vi "2015Swerve.vi"(0 "Axes":dbl[](array[numeric]), 2 "Robot Dimension Calc":dbl, 4 "EncoderTicksPerRev":dbl, 6 "Encoder Offset":dbl) -> (20 "SteeringArray":dbl[](array[numeric]), 22 "PowerArray":dbl[](array[numeric]))   [LabVIEW 2014]
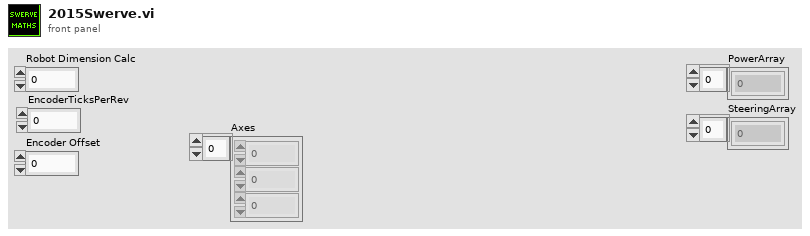
[diagram p1: front panel]
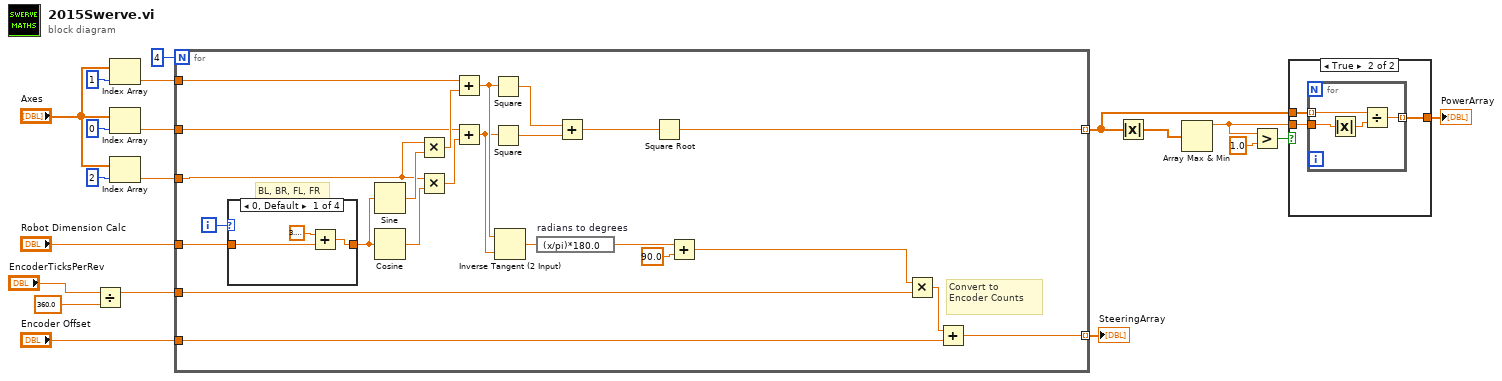
[diagram p0: block diagram]
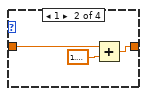
[diagram p3: hidden frame]
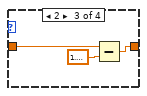
[diagram p4: hidden frame]
diagram:
  n1 = Divide(x="EncoderTicksPerRev", y=360.0) -> (x/y=w5:dbl)
  n2 = Index Array(array="Axes", index=1) -> (element=w9:dbl)
  n3 = Index Array(array="Axes", index=0) -> (element=w10:dbl)
  n4 = Index Array(array="Axes", index=2) -> (element=w11:dbl)
  n5 = for {
    N: 4 -> [_]
    tunnel: "Robot Dimension Calc" -> [w44]
    tunnel: w11 -> [w23]
    tunnel: w10 -> [w22]
    tunnel: w9 -> [w21]
    tunnel: [w27] -> w1 mode=indexing
    tunnel: [w25] -> w15 mode=indexing
    tunnel: w5 -> [w29]
    tunnel: "Encoder Offset" -> [w26]
    i -> [w39]
    # "Convert to\nEncoder Counts"
    # "BL, BR, FL, FR"
    n6 = case shown="0, Default" w39 {
      tunnel: [w46 w50 w53 w54] -> w30
      tunnel: w44 -> [w47 w48 w51 w54]
      frame 0, Default {
        n7 = Add(x=3.141592653589793, y=w47) -> (x+y=w46:dbl)
      }
      frame 1 {
        n8 = Add(x=w48, y=1.5707963267948966) -> (x+y=w50:dbl)
      }
      frame 2 {
        n9 = Subtract(x=w51, y=1.5707963267948966) -> (x-y=w53:dbl)
      }
      frame 3 {
      }
    }
    n10 = Sine(x=w30) -> (sin(x)=w42:dbl)
    n11 = Cosine(x=w30) -> (cos(x)=w43:dbl)
    n12 = Multiply(x=w23, y=w42) -> (x*y=w33:dbl)
    n13 = Multiply(x=w23, y=w43) -> (x*y=w41:dbl)
    n14 = Add(x=w21, y=w33) -> (x+y=w38:dbl)
    n15 = Add(x=w22, y=w41) -> (x+y=w34:dbl)
    n16 = Square(x=w38) -> (x^2=w37:dbl)
    n17 = Square(x=w34) -> (x^2=w36:dbl)
    n18 = Inverse Tangent (2 Input)(1:w34, 2:w38) -> (0:w40:dbl)
    n19 = expression code="(x/pi)*180.0" "radians to degrees"(w40) -> (w32:dbl)
    n20 = Add(x=w37, y=w36) -> (x+y=w35:dbl)
    n21 = Square Root(x=w35) -> (sqrt(x)=w25:dbl)
    n22 = Add(x=w32, y=90.0) -> (x+y=w24:dbl)
    n23 = Multiply(x=w24, y=w29) -> (x*y=w28:dbl)
    n24 = Add(x=w28, y=w26) -> (x+y=w27:dbl)
  }
  "SteeringArray" <- w1
  n25 = Absolute Value(x=w15) -> (abs(x)=w19:dbl[])
  n26 = Array Max & Min(array=w19) -> (max value=w17:dbl)  [unwired: 3 out]
  n27 = Greater?(x=w17, y=1.0) -> (0:w16:bool)
  n28 = case shown="True" w16 {
    tunnel: w15 -> [w55 w58]
    tunnel: w17 -> [_ w57]
    tunnel: [w55 w56] -> w2
    frame False {
    }
    frame True {
      n29 = for {
        tunnel: w58 -> [w62] mode=indexing
        tunnel: w57 -> [w60]
        tunnel: [w59] -> w56 mode=indexing
        n30 = Absolute Value(x=w60) -> (abs(x)=w61:dbl)
        n31 = Divide(x=w62, y=w61) -> (x/y=w59:dbl)
      }
    }
  }
  "PowerArray" <- w2
